vi "ATF-Sequence Files Seperater.vi"(10 "Array in":string[](array[string]), 11 "Sequence":path) -> (3 "Array":T1(array[cluster]))   [LabVIEW 2022 SP3]
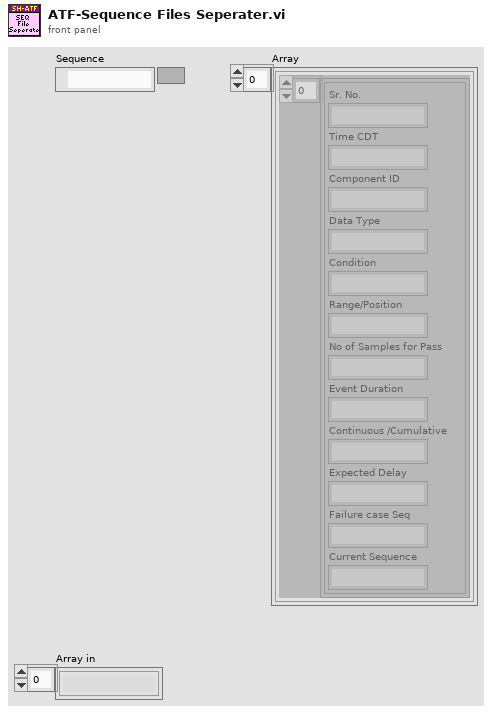
[diagram p1: front panel]
types:
  T1 = cluster{cluster{"Sr. No.":string, "Time CDT":string, "Component ID":string, "Data Type":string, "Condition":string, "Range/Position":string, "No of Samples for Pass":string, "Event Duration":string, "Continuous /Cumulative":string, "Expected Delay":string, "Failure case Seq":string, "Current Sequence":string}[]}[]
  T2 = cluster{"Sr. No.":string, "Time CDT":string, "Component ID":string, "Data Type":string, "Condition":string, "Range/Position":string, "No of Samples for Pass":string, "Event Duration":string, "Continuous /Cumulative":string, "Expected Delay":string, "Failure case Seq":string, "Current Sequence":string}[]
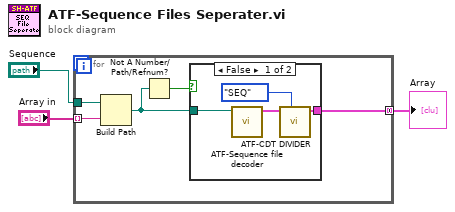
[diagram p0: block diagram]
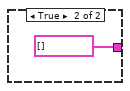
[diagram p2: hidden frame]
diagram:
  n1 = for {
    tunnel: "Array in" -> [w8] mode=indexing
    tunnel: "Sequence" -> [w7]
    tunnel: [w6] -> w3 mode=concatenating
    n2 = Build Path(base path=w7, name or relative path=w8) -> (appended path=w4:path)
    n3 = Not A Number/Path/Refnum?(number/path/refnum=w4) -> (NaN/Path/Refnum?=w5:bool)
    n4 = case shown="False" w5 {
      tunnel: w4 -> [w12 _]
      tunnel: [w9 T1 [] ("Array")] -> w6
      frame False {
        n5 = call "ATF-Sequence file decoder.vi"("file path (dialog if empty)"=w12) -> ("Seq in"=w10:T2)  [unwired: 9 in, 1 out]
        n6 = call "ATF-CDT DIVIDER.vi"("Enum"=enum16{"SEQ", "CDT"}."SEQ", "Seq in"=w10) -> ("Array"=w9:T1)  [unwired: 9 in]
      }
      frame True {
      }
    }
  }
  "Array" <- w3
